vi "read Configuration Ver3.vi"(10 "pseudoPdcId":i32, 11 "timeoutMs":i32) -> (3 "function return":i32)   [LabVIEW 2013, in "C37118-DLL.lvlib" / "StrongridDLL.lvlib"]
doc: "STRONGRIDIEEEC37118DLL_API int __cdecl readConfiguration_Ver3( int32_t timeoutMs, int32_t pseudoPdcId);"
uses:
  StrongridDLL.lvlib
  <vilib>/S3DK/data/StrongridDLL.dll
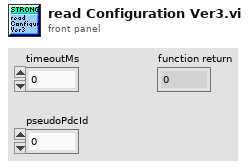
[diagram p1: front panel]
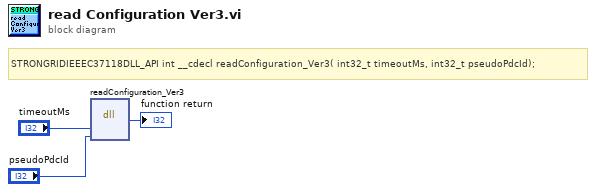
[diagram p0: block diagram]
diagram:
  # "STRONGRIDIEEEC37118DLL_API int __cdecl readConfiguration_Ver3( int32_t timeoutMs, int32_t pseudoPdcId);"
  n1 = dll-call lib="C:/Program Files (x86)/National Instruments/LabVIEW 2013/vi.lib/S3DK/data/StrongridDLL.*" fn="readConfiguration_Ver3"("timeoutMs"="timeoutMs", "pseudoPdcId"="pseudoPdcId") -> (→"function return":i32)  [unwired: 5 in, 2 out]
